vi "Alterrum.vi"() -> ()   [LabVIEW 2020]
uses:
  Type Definitions/Computer Metadata.ctl
  Type Definitions/Internet Connection Monitor.ctl
  Type Definitions/CPU Usage.ctl
  Type Definitions/Disk State.ctl
  Type Definitions/Memory Monitor.ctl
  Type Definitions/System Time.ctl
  Type Definitions/Data Frame.ctl
  Type Definitions/Data Frame Header.ctl
  Type Definitions/Payload Class.ctl
  Type Definitions/Telemetry TCP State.ctl
  Type Definitions/Telemetry Recorder Status.ctl
  Type Definitions/Queue Monitor.ctl
  Type Definitions/RTOSMonitor.ctl
  Type Definitions/Command TCP State.ctl
  Type Definitions/Notification Data.ctl
  Type Definitions/Enum - Notification Types.ctl
  Type Definitions/Network Adapter State.ctl
  Type Definitions/Discovery Engine State.ctl
  Type Definitions/Analog Output Command.ctl
  Type Definitions/Digital Output Command.ctl
  Type Definitions/Digital Output Data.ctl
  Type Definitions/Analog Input Data.ctl
  Type Definitions/Analog Output Data.ctl
  <vilib>/ptbypt/NI_PtbyPt.lvlib
panel:
  out "Command IP Address":string
  out "Telemetry IP Address":string
  out "Detected IP Addresses":string[](array[string])
  out "Telemetry Handler":T1 {"CRC" format="%08x"; "Frame Header"."Options" format="%016b"; "Frame Header"."Time" format="%<%I:%M:%S%3u %p\n%m/%d/%Y>T"; "Frame Header"."Sync" format="%08x"}
  in  "Main Tabs":T4(tab)
  out "Computer Metadata":T5
  out "CPU Utilization":dbl[][](graph)
  out "Available Memory":dbl[][](graph)
  out "Internet Connection Monitor":T6
  out "CPU Monitor":T7 {"Idle CPU Time" format="%#.2f"; "SIRQ CPU Usage" format="%#.2f"; "IRQ CPU Usage" format="%#.2f"; "IO CPU Usage" format="%#.2f"; "NIC CPU" format="%#.2f"; "System CPU Usage" format="%#.2f"; "User CPU Usage" format="%#.2f"}
  out "Memory Monitor":T8 {"Available Memory" format="%#.2f"; "Total Memory" format="%#.2f"}
  out "RTOS Monitor":T9[](array[typedef])
  out "Archive Monitor":T10
  out "Queue Monitor":T11[](array[typedef])
  out "System Time":T12
  out "Telemetry TCP State":T13
  out "Command TCP State":T14
  out "Network Adapter State":T15
  out "Discovery Engine State":T16[](array[typedef])
  out "Disk Management":T17[](array[typedef]) {"Used" format="%#.2f"; "Available" format="%#.2f"; "Total" format="%#.2f"}
  out "Analog Output Data":dbl[][](graph)
  out "Analog Input Data":dbl[][](graph)
  out "Notification Data":cluster{"Time":dbl, T18} {"Time" format="%<%I:%M:%S%3u %p\n%m/%d/%Y>T"}
  in  "Analog Output Command":T20 {"State" scale=0.0..5.0}
  in  "Send Analog Command":bool
  in  "Send Digital Command":bool
  in  "Digital Output Command":T21
  in  "Null Command":bool
  out "Command Ack":T1 {"CRC" format="%08x"; "Frame Header"."Options" format="%016b"; "Frame Header"."Time" format="%<%I:%M:%S%3u %p\n%m/%d/%Y>T"; "Frame Header"."Sync" format="%08x"}
  out "Digital Output Data":T22 {"Port 0" format="%08b"}
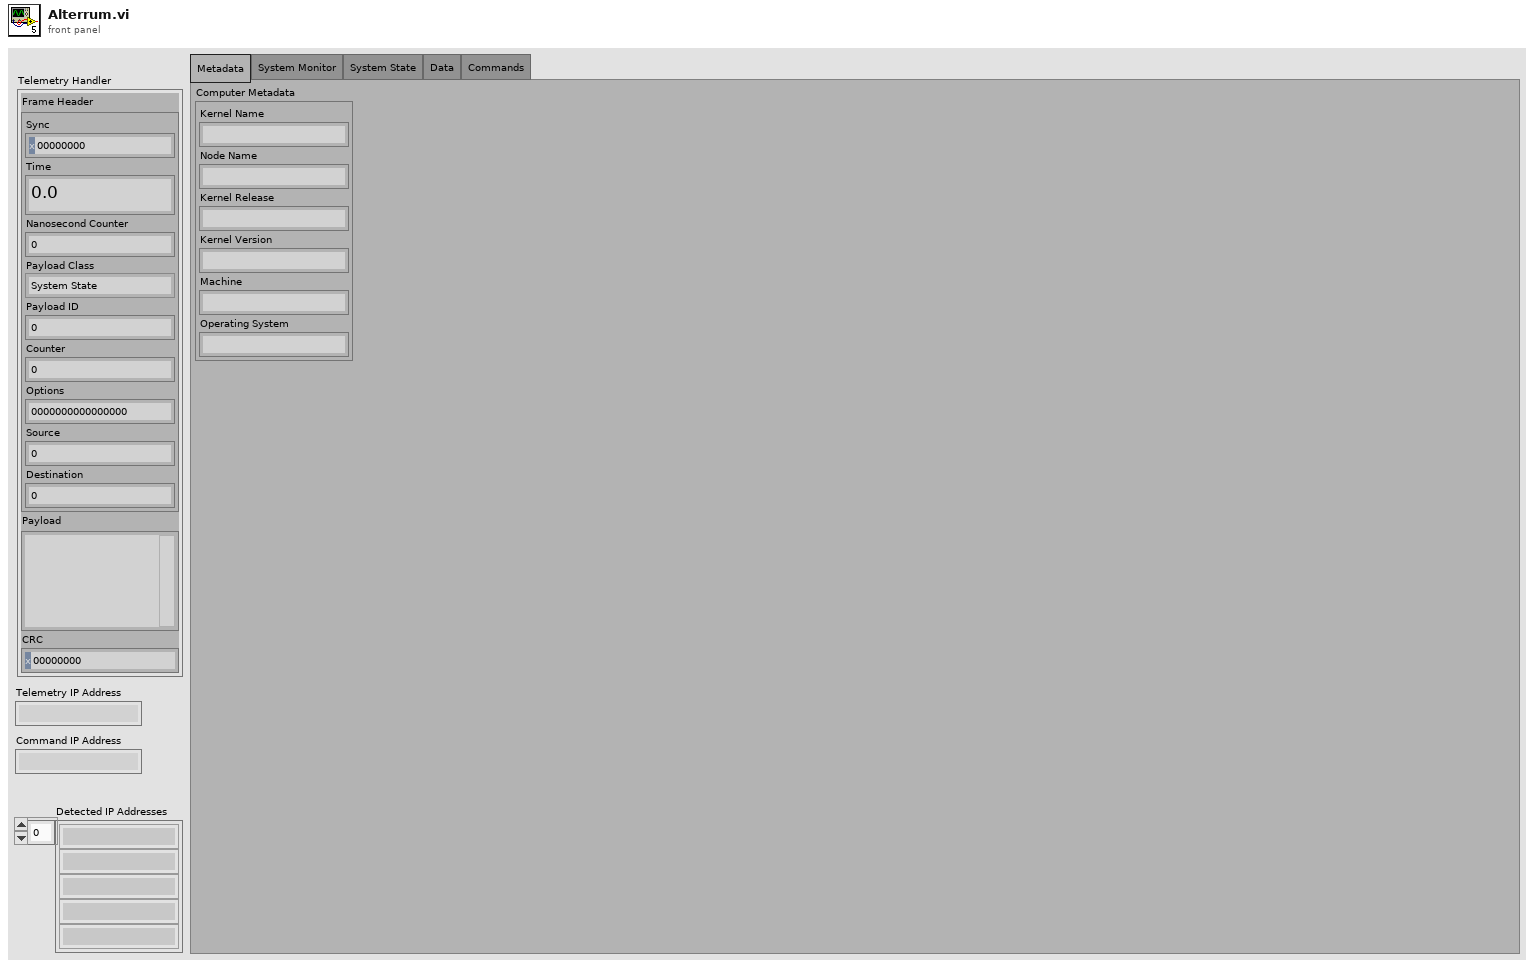
[diagram p1: front panel]
types:
  T1 = typedef "Data Frame.ctl" = cluster{"Frame Header":T2, "Payload":string, "CRC":u32}
  T2 = typedef "Data Frame Header.ctl" = cluster{"Sync":u32, "Time":dbl, "Nanosecond Counter":i64, "Payload Class":T3, "Payload ID":u16, "Counter":u32, "Options":u32, "Source":i32, "Destination":i32}
  T3 = typedef "Payload Class.ctl" = enum16{"System State", "Parameters", "Metadata", "Software Monitor", "Data", "Commands"}
  T4 = enum32{"Metadata", "System Monitor", "System State", "Data", "Commands"}
  T5 = typedef "Computer Metadata.ctl" = cluster{"Kernel Name":string, "Node Name":string, "Kernel Release":string, "Kernel Version":string, "Machine":string, "Operating System":string}
  T6 = typedef "Internet Connection Monitor.ctl" = cluster{"Connected?":bool, "Ping Latency (uS)":i32, "Ping Address":string}
  T7 = typedef "CPU Usage.ctl" = cluster{"User CPU Usage":sgl, "System CPU Usage":sgl, "NIC CPU ":sgl, "IO CPU Usage":sgl, "IRQ CPU Usage":sgl, "SIRQ CPU Usage":sgl, "Idle CPU Time":sgl}
  T8 = typedef "Memory Monitor.ctl" = cluster{"Total Memory":sgl, "Available Memory":sgl}
  T9 = typedef "RTOSMonitor.ctl" = cluster{"Task Name":string, "Priority":i32, "Processor":i32, "Offset":i64, "Min Duration":i64, "Mean Duration":i64, "Max Duration":i64, "Period":i64, "Late Iterations":i16, "Iteration Count":i32}
  T10 = typedef "Telemetry Recorder Status.ctl" = cluster{"Filepath":string, "File Size":i64, "Frame Count":i32, "Mean MB/hour":sgl}
  T11 = typedef "Queue Monitor.ctl" = cluster{"Queue Name":string, "Max Queue Size":i32, "Pending Remove":i32, "Pending Insert":i32, "Elements in Queue":i32}
  T12 = typedef "System Time.ctl" = cluster{"System Time":timestamp, "Get Date/Time":timestamp, "Microsecond Clock":i64}
  T13 = typedef "Telemetry TCP State.ctl" = cluster{"Is Connected":bool, "Remote Address":string, "Remote Port":u16, "Total Frames Sent":i32, "Total Bytes Sent":i32}
  T14 = typedef "Command TCP State.ctl" = cluster{"Is Connected":bool, "Remote Address":string, "Remote Port":u16, "Total Frames Sent":i32, "Total Bytes Sent":i32}
  T15 = typedef "Network Adapter State.ctl" = cluster{"Adapter IP Addresses":string[]}
  T16 = typedef "Discovery Engine State.ctl" = cluster{"Adapter IP Address":string, "Connection ID":refnum<k16>, "Error":errorcluster}
  T17 = typedef "Disk State.ctl" = cluster{"File System Name":string, "Total":sgl, "Available":sgl, "Used":sgl, "Path":string}
  T18 = typedef "Notification Data.ctl" = cluster{"Notification Type":T19, "Code":i32, "Description":string}
  T19 = typedef "Enum - Notification Types.ctl" = enum16{"Warning", "Acknowledge", "Notification"}
  T20 = typedef "Analog Output Command.ctl" = cluster{"AO Channel":u8, "State":dbl}
  T21 = typedef "Digital Output Command.ctl" = cluster{"DO Channel":u8, "State":bool}
  T22 = typedef "Digital Output Data.ctl" = cluster{"Port 0":u8}
  T23 = typedef "Analog Input Data.ctl" = cluster{"Analog Data":dbl[][]}
  T24 = typedef "Analog Output Data.ctl" = cluster{"Bank 0":dbl[]}
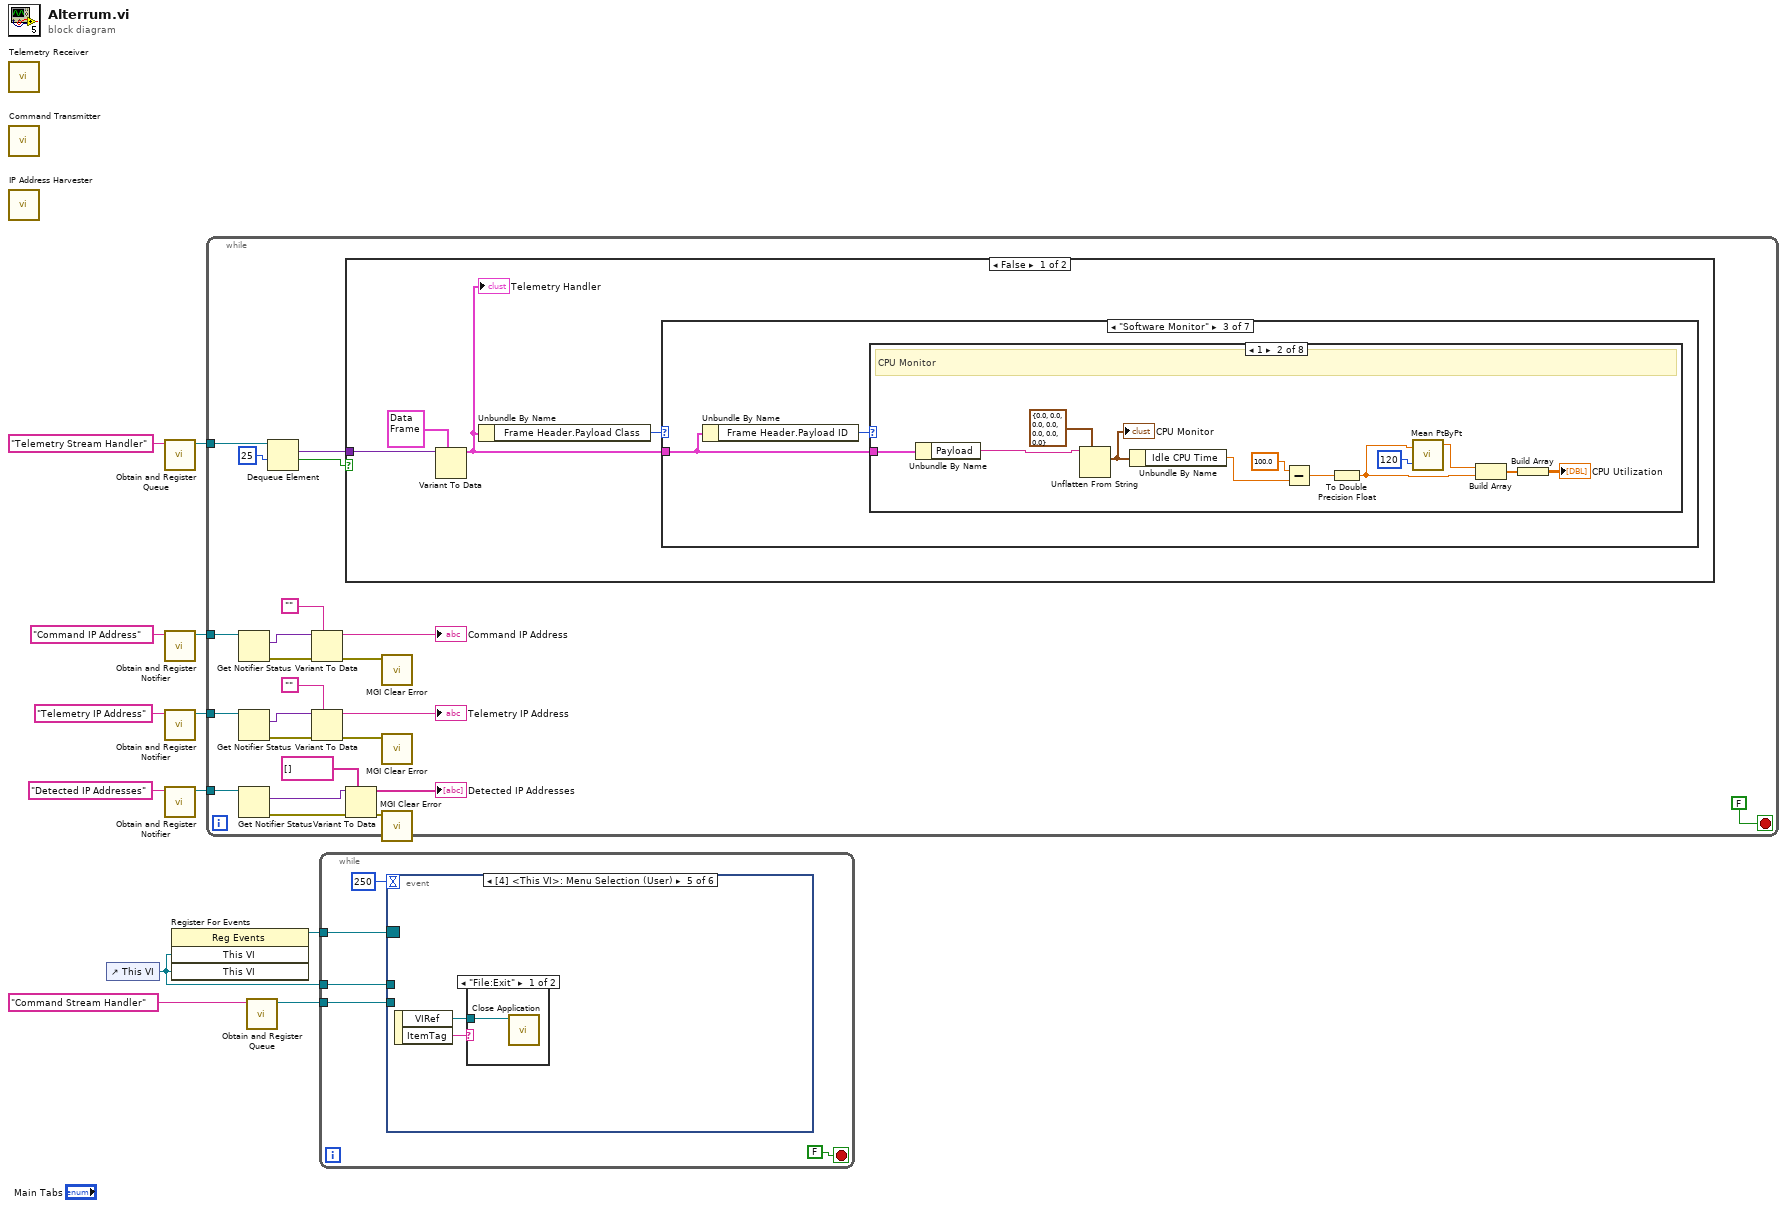
[diagram p0: block diagram]
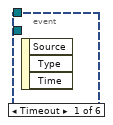
[diagram p2: hidden frame]
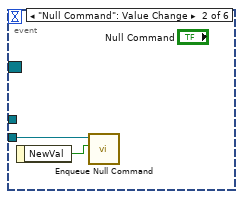
[diagram p3: hidden frame]
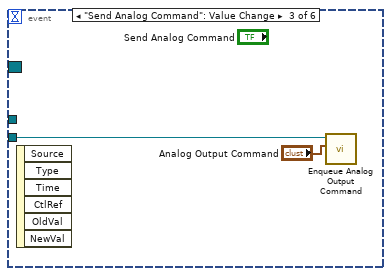
[diagram p4: hidden frame]
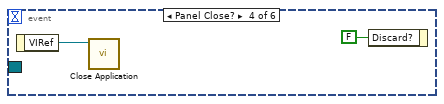
[diagram p5: hidden frame]
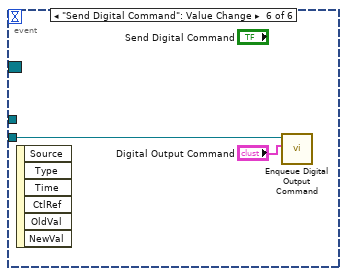
[diagram p7: hidden frame]
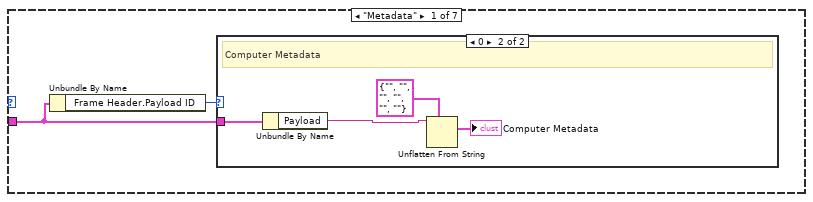
[diagram p8: hidden frame]
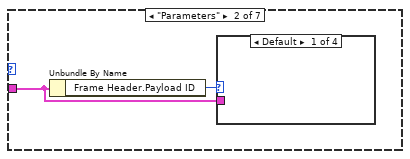
[diagram p10: hidden frame]
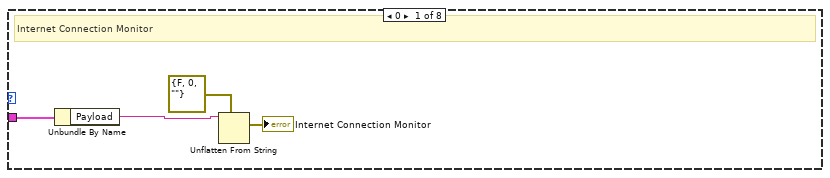
[diagram p14: hidden frame]
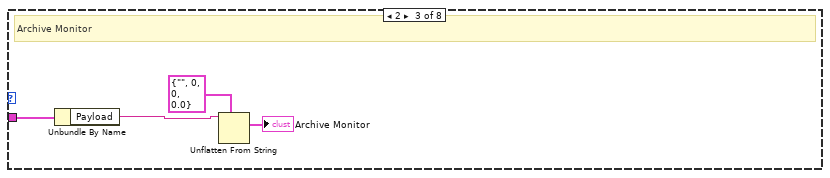
[diagram p15: hidden frame]
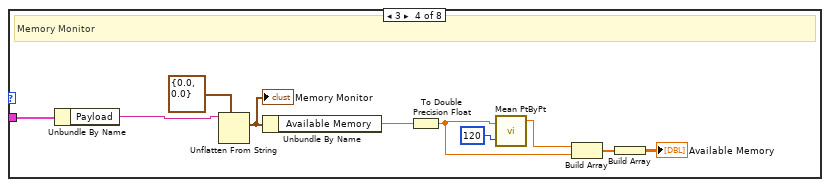
[diagram p16: hidden frame]
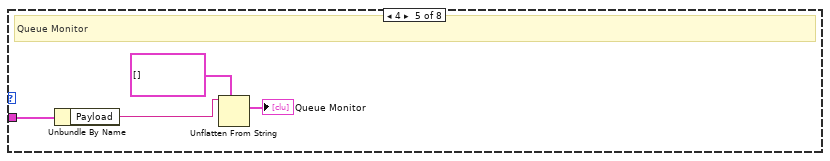
[diagram p17: hidden frame]
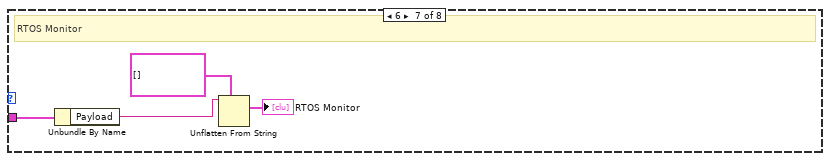
[diagram p19: hidden frame]
diagram:
  n1 = call "Telemetry Receiver.vi"() -> ()  [unwired: 12 in]
  n2 = call "Command Transmitter.vi"() -> ()  [unwired: 12 in]
  n3 = call "IP Address Harvester.vi"() -> ()  [unwired: 12 in]
  n4 = control-ref of="This VI"() -> (w9:refnum<vi>)
  n5 = call "Obtain and Register Queue.vi"("name (unnamed)"="Telemetry Stream Handler") -> ("Queue Out"=w11:refnum<queue>)  [unwired: 7 in, 3 out]
  n6 = call "Obtain and Register Notifier.vi"("name (unnamed)"="Command IP Address") -> ("notifier out"=w1:refnum<notifier>)  [unwired: 8 in, 2 out]
  n7 = call "Obtain and Register Notifier.vi"("name (unnamed)"="Telemetry IP Address") -> ("notifier out"=w3:refnum<notifier>)  [unwired: 8 in, 2 out]
  n8 = call "Obtain and Register Notifier.vi"("name (unnamed)"="Detected IP Addresses") -> ("notifier out"=w2:refnum<notifier>)  [unwired: 8 in, 2 out]
  n9 = register-events(w9, w9) -> (reference out=w10:refnum<event-registration>)  [unwired: 2 in, 1 out]
  n10 = while {
    tunnel: w11 -> [w34]
    tunnel: w3 -> [w19]
    tunnel: w2 -> [w16]
    tunnel: w1 -> [w15]
    stop <- FALSE stop-if-true
    n11 = Get Notifier Status(notifier=w15) -> (current notification=w21:variant, error out=w24:errorcluster)  [unwired: 1 in, 3 out]
    n12 = Get Notifier Status(notifier=w19) -> (current notification=w29:variant, error out=w28:errorcluster)  [unwired: 1 in, 3 out]
    n13 = Get Notifier Status(notifier=w16) -> (current notification=w23:variant, error out=w26:errorcluster)  [unwired: 1 in, 3 out]
    n14 = Dequeue Element(queue=w34, timeout in ms (-1)=25) -> (element=w35:variant, timed out?=w31:bool)  [unwired: 1 in, 2 out]
    n15 = Variant To Data(error in=w24, type="", Variant=w21) -> (data=→"Command IP Address":string, error out=w25:errorcluster)
    n16 = Variant To Data(error in=w28, type="", Variant=w29) -> (data=→"Telemetry IP Address":string, error out=w13:errorcluster)
    n17 = case shown="False" w31 {
      tunnel: w35 -> [w38 _]
      frame False {
        n18 = Variant To Data(type=T1 {"Frame Header"={"Sync"=0, "Time"=0.0, "Nanosecond Counter"=0, "Payload Class"=enum."System State", "Payload ID"=0, "Counter"=0, "Options"=0, "Source"=0, "Destination"=0}, "Payload"="", "CRC"=0} ("Frame"), Variant=w38) -> (data=w36:T1)  [unwired: 1 in, 1 out]
        "Telemetry Handler" <- w36
        n19 = Unbundle By Name(w36) -> ("Frame Header.Payload Class"=w39:T3)
        n20 = case shown="\"Software Monitor\"" w39 {
          tunnel: w36 -> [w40 w46 w49 w88 w114 _ _]
          frame "Metadata" {
            n21 = Unbundle By Name(w40) -> ("Frame Header.Payload ID"=w41:u16)
            n22 = case shown="0" w41 {
              tunnel: w40 -> [_ w45]
              frame Default {
              }
              frame 0 {
                # "Computer Metadata"
                n23 = Unbundle By Name(w45) -> ("Payload"=w44:string)
                n24 = Unflatten From String(type=T5 {"Kernel Name"="", "Node Name"="", "Kernel Release"="", "Kernel Version"="", "Machine"="", "Operating System"=""} ("Computer Metadata"), binary string=w44) -> (value=→"Computer Metadata":T5)  [unwired: 3 in, 2 out]
              }
            }
          }
          frame "Parameters" {
            n25 = Unbundle By Name(w46) -> ("Frame Header.Payload ID"=w47:u16)
            n26 = case shown="Default" w47 {
              tunnel: w46 -> [_ _ _ _]
              frame Default {
              }
              frame 0 {
              }
              frame 1 {
              }
              frame 2 {
              }
            }
          }
          frame "Software Monitor" {
            n27 = Unbundle By Name(w49) -> ("Frame Header.Payload ID"=w48:u16)
            n28 = case shown="1" w48 {
              tunnel: w49 -> [w53 w65 w66 w79 w80 _ w86 _]
              frame 0 {
                # "Internet Connection Monitor"
                n29 = Unbundle By Name(w53) -> ("Payload"=w52:string)
                n30 = Unflatten From String(type=T6 {"Connected?"=FALSE, "Ping Latency (uS)"=0, "Ping Address"=""} ("Internet Connection Monitor"), binary string=w52) -> (value=→"Internet Connection Monitor":T6)  [unwired: 3 in, 2 out]
              }
              frame 1 {
                # "CPU Monitor"
                n31 = Unbundle By Name(w65) -> ("Payload"=w64:string)
                n32 = Unflatten From String(type=T7 {"User CPU Usage"=0.0, "System CPU Usage"=0.0, "NIC CPU "=0.0, "IO CPU Usage"=0.0, "IRQ CPU Usage"=0.0, "SIRQ CPU Usage"=0.0, "Idle CPU Time"=0.0}, binary string=w64) -> (value=w62:T7)  [unwired: 3 in, 2 out]
                "CPU Monitor" <- w62
                n33 = Unbundle By Name(w62) -> ("Idle CPU Time"=w61:sgl)
                n34 = Subtract(x=sgl 100.0 ("y"), y=w61) -> (x-y=w57:sgl)
                n35 = To Double Precision Float(number=w57) -> (double precision float=w56:dbl)
                n36 = call <vilib>:"Mean PtByPt.vi"("x"=w56, "sample length"=120) -> ("mean"=w58:dbl)  [unwired: 2 in, 1 out]
                n37 = Build Array(w58, w56) -> (w55:dbl[])
                n38 = Build Array(w55) -> (→"CPU Utilization":dbl[][])
              }
              frame 2 {
                # "Archive Monitor"
                n39 = Unbundle By Name(w66) -> ("Payload"=w68:string)
                n40 = Unflatten From String(type=T10 {"Filepath"="", "File Size"=0, "Frame Count"=0, "Mean MB/hour"=0.0}, binary string=w68) -> (value=→"Archive Monitor":T10)  [unwired: 3 in, 2 out]
              }
              frame 3 {
                # "Memory Monitor"
                n41 = Unbundle By Name(w79) -> ("Payload"=w78:string)
                n42 = Unflatten From String(type=T8 {"Total Memory"=0.0, "Available Memory"=0.0}, binary string=w78) -> (value=w76:T8)  [unwired: 3 in, 2 out]
                "Memory Monitor" <- w76
                n43 = Unbundle By Name(w76) -> ("Available Memory"=w73:sgl)
                n44 = To Double Precision Float(number=w73) -> (double precision float=w72:dbl)
                n45 = call <vilib>:"Mean PtByPt.vi"("x"=w72, "sample length"=120) -> ("mean"=w74:dbl)  [unwired: 2 in, 1 out]
                n46 = Build Array(w74, w72) -> (w71:dbl[])
                n47 = Build Array(w71) -> (→"Available Memory":dbl[][])
              }
              frame 4 {
                # "Queue Monitor"
                n48 = Unbundle By Name(w80) -> ("Payload"=w83:string)
                n49 = Unflatten From String(type=T11[] [] ("cluster"), binary string=w83) -> (value=→"Queue Monitor":T11[])  [unwired: 3 in, 2 out]
              }
              frame 5 {
                # "RTOS Update - Not Transmitted"
              }
              frame 6 {
                # "RTOS Monitor"
                n50 = Unbundle By Name(w86) -> ("Payload"=w87:string)
                n51 = Unflatten From String(type=T9[] [] ("cluster"), binary string=w87) -> (value=→"RTOS Monitor":T9[])  [unwired: 3 in, 2 out]
              }
              frame Default {
              }
            }
          }
          frame "System State" {
            n52 = Unbundle By Name(w88) -> ("Frame Header.Payload ID"=w89:u16)
            n53 = case shown="3" w89 {
              tunnel: w88 -> [w93 w97 _ w101 w105 w109 w110 _]
              frame 0 {
                # "System Time"
                n54 = Unbundle By Name(w93) -> ("Payload"=w92:string)
                n55 = Unflatten From String(type=T12 {"System Time"=timestamp(0 s since 1904-01-01), "Get Date/Time"=timestamp(0 s since 1904-01-01), "Microsecond Clock"=0}, binary string=w92) -> (value=→"System Time":T12)  [unwired: 3 in, 2 out]
              }
              frame 1 {
                # "Telemetry TCP State"
                n56 = Unbundle By Name(w97) -> ("Payload"=w96:string)
                n57 = Unflatten From String(type=T13 {"Is Connected"=FALSE, "Remote Address"="", "Remote Port"=0, "Total Frames Sent"=0, "Total Bytes Sent"=0} ("Cluster"), binary string=w96) -> (value=→"Telemetry TCP State":T13)  [unwired: 3 in, 2 out]
              }
              frame 2 {
                # "Writeable Drive State - Inactive"
              }
              frame 3 {
                # "Command TCP State"
                n58 = Unbundle By Name(w101) -> ("Payload"=w100:string)
                n59 = Unflatten From String(type=T14 {"Is Connected"=FALSE, "Remote Address"="", "Remote Port"=0, "Total Frames Sent"=0, "Total Bytes Sent"=0} ("Network Stream Status"), binary string=w100) -> (value=→"Command TCP State":T14)  [unwired: 3 in, 2 out]
              }
              frame 4 {
                # "Network Adapter State"
                n60 = Unbundle By Name(w105) -> ("Payload"=w104:string)
                n61 = Unflatten From String(type=T15 {"Adapter IP Addresses"=[]}, binary string=w104) -> (value=→"Network Adapter State":T15)  [unwired: 3 in, 2 out]
              }
              frame 5 {
                # "Discovery Engine State"
                n62 = Unbundle By Name(w109) -> ("Payload"=w108:string)
                n63 = Unflatten From String(type=T16[] [] ("Array"), binary string=w108) -> (value=→"Discovery Engine State":T16[])  [unwired: 3 in, 2 out]
              }
              frame 6 {
                # "Disk State"
                n64 = Unbundle By Name(w110) -> ("Payload"=w113:string)
                n65 = Unflatten From String(type=T17[] [], binary string=w113) -> (value=→"Disk Management":T17[])  [unwired: 3 in, 2 out]
              }
              frame Default {
              }
            }
          }
          frame "Data" {
            n66 = Unbundle By Name(w114) -> ("Frame Header.Payload ID"=w115:u16)
            n67 = case shown="0" w115 {
              tunnel: w114 -> [_ w120 w126 w132 w136 w140]
              frame Default {
              }
              frame 0 {
                # "Analog Input Data"
                n68 = Unbundle By Name(w120) -> ("Payload"=w119:string)
                n69 = Unflatten From String(type=T23 {"Analog Data"=[]}, binary string=w119) -> (value=w117:T23)  [unwired: 3 in, 2 out]
                n70 = Unbundle By Name(w117) -> ("Analog Data"=→"Analog Input Data":dbl[][])
              }
              frame 1 {
                # "Notification Data"
                n71 = Unbundle By Name(w126) -> ("Frame Header.Time"=w123:dbl, "Payload"=w125:string)
                n72 = Unflatten From String(type=T18 {"Notification Type"=enum."Warning", "Code"=0, "Description"=""}, binary string=w125) -> (value=w122:T18)  [unwired: 3 in, 2 out]
                n73 = Bundle("Time"=w123, w122) -> (→"Notification Data":cluster{"Time":dbl, T18})  [unwired: 1 in]
              }
              frame 2 {
                # "Analog Output Data"
                n74 = Unbundle By Name(w132) -> ("Payload"=w131:string)
                n75 = Unflatten From String(type=T24 {"Bank 0"=[]}, binary string=w131) -> (value=w128:T24)  [unwired: 3 in, 2 out]
                n76 = Unbundle By Name(w128) -> ("Bank 0"=w127:dbl[])
                n77 = Build Array(w127) -> (→"Analog Output Data":dbl[][])
              }
              frame 3 {
                # "Digital Output Data"
                n78 = Unbundle By Name(w136) -> ("Payload"=w135:string)
                n79 = Unflatten From String(type=T22 {"Port 0"=0}, binary string=w135) -> (value=→"Digital Output Data":T22)  [unwired: 3 in, 2 out]
              }
              frame 4 {
                # "Command Ack"
                n80 = Unbundle By Name(w140) -> ("Payload"=w139:string)
                n81 = Unflatten From String(type=T1 {"Frame Header"={"Sync"=0, "Time"=0.0, "Nanosecond Counter"=0, "Payload Class"=enum."System State", "Payload ID"=0, "Counter"=0, "Options"=0, "Source"=0, "Destination"=0}, "Payload"="", "CRC"=0} ("Frame"), binary string=w139) -> (value=→"Command Ack":T1)  [unwired: 3 in, 2 out]
              }
            }
          }
          frame "Commands" {
          }
          frame Default {
          }
        }
      }
      frame True {
      }
    }
    n82 = Variant To Data(error in=w26, type=string[] [] ("Adapter IP Addresses"), Variant=w23) -> (data=→"Detected IP Addresses":string[], error out=w27:errorcluster)
    n83 = call <userlib>:"MGI Clear Error.vi"("Error In"=w25) -> ()  [unwired: 6 in, 1 out]
    n84 = call <userlib>:"MGI Clear Error.vi"("Error In"=w13) -> ()  [unwired: 6 in, 1 out]
    n85 = call <userlib>:"MGI Clear Error.vi"("Error In"=w27) -> ()  [unwired: 6 in, 1 out]
  }
  n86 = call "Obtain and Register Queue.vi"("name (unnamed)"="Command Stream Handler") -> ("Queue Out"=w7:refnum<queue>)  [unwired: 7 in, 3 out]
  n87 = while {
    tunnel: w7 -> [w144]
    tunnel: w10 -> [w143]
    tunnel: w9 -> [w142]
    stop <- FALSE stop-if-true
    n88 = event shown="[4] <This VI>: Menu Selection (User)" {
      selector: w143 -> [_ _ _ _ _ _]
      dyn-events: _ -> [_ _ _ _ _ _]
      timeout: 250 -> [_ _ _ _ _ _]
      tunnel: w144 -> [_ w147 w149 _ _ w156]
      tunnel: w142 -> [_ _ _ _ _ _]
      event Timeout {
        n89 = event-data() -> ()  [unwired: 1 in, 3 out]
      }
      event "Null Command": Value Change {
        n90 = event-data() -> ("NewVal"=w146:bool)  [unwired: 1 in]
        n91 = call "Enqueue Null Command.vi"("NewVal"=w146, "Queue in"=w147) -> ()  [unwired: 10 in]
      }
      event "Send Analog Command": Value Change {
        n92 = event-data() -> ()  [unwired: 1 in, 6 out]
        n93 = call "Enqueue Analog Output Command.vi"("Analog Output Command"="Analog Output Command", "Queue In"=w149) -> ()  [unwired: 10 in]
      }
      event Panel Close? {
        n94 = event-data() -> ("VIRef"=w150:refnum<vi>)  [unwired: 1 in]
        n95 = call "Close Application.vi"("VI in"=w150) -> ()  [unwired: 11 in]
        n96 = event-data("Discard?"=FALSE) -> ()  [unwired: 1 in, 1 out]
      }
      event Menu Selection (User) {
        n97 = event-data() -> ("VIRef"=w152:refnum<vi>, "ItemTag"=w153:string)  [unwired: 1 in]
        n98 = case shown="\"File:Exit\"" w153 {
          tunnel: w152 -> [w154 _]
          frame "File:Exit" {
            n99 = call "Close Application.vi"("VI in"=w154) -> ()  [unwired: 11 in]
          }
          frame Default {
          }
        }
      }
      event "Send Digital Command": Value Change {
        n100 = event-data() -> ()  [unwired: 1 in, 6 out]
        n101 = call "Enqueue Digital Output Command.vi"("Digital Output Command"="Digital Output Command", "Queue In"=w156) -> ()  [unwired: 10 in]
      }
    }
  }
